vi "Read Unparsed Metadata from TDMS.vi"(8 "error in (no error)":errorcluster, 11 "file path":path) -> (0 "error out":errorcluster, 2 "sweepctl json":string, 3 "yaml metadata":string)   [LabVIEW 2016]
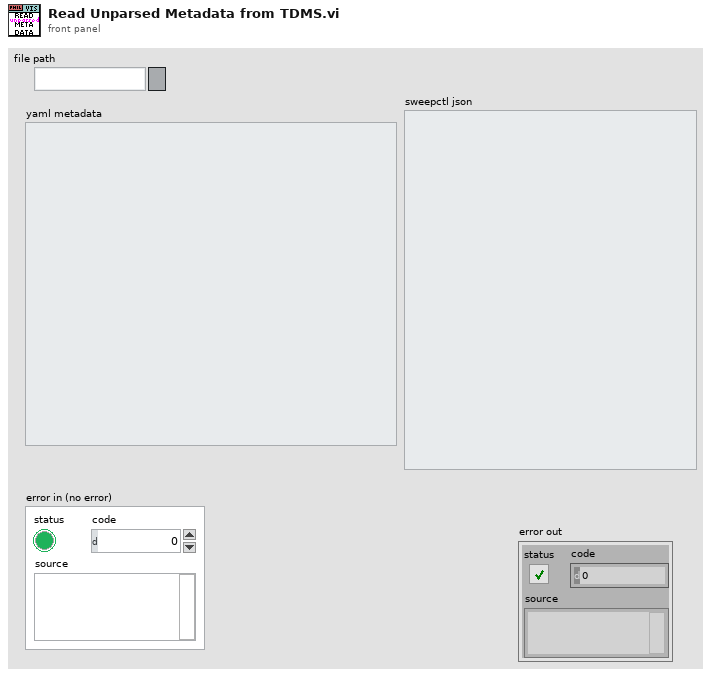
[diagram p1: front panel]
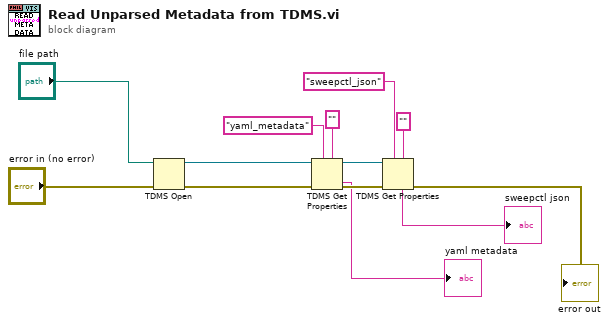
[diagram p0: block diagram]
diagram:
  n1 = TDMS Open(8:"error in (no error)", 11:"file path") -> (0:w10:errorcluster, 3:w11:refnum<k34>)  [unwired: 5 in]
  n2 = TDMS Get Properties(5:"", 7:"yaml_metadata", 8:w10, 11:w11) -> (0:w7:errorcluster, 3:w6:refnum<k34>, 4:→"yaml metadata":string)  [unwired: 2 in, 3 out]
  n3 = TDMS Get Properties(5:"", 7:"sweepctl_json", 8:w7, 11:w6) -> (0:→"error out":errorcluster, 4:→"sweepctl json":string)  [unwired: 2 in, 4 out]
